vi "CLC_L2_8x8_InPhaseCal_L1_2x2.vi"() -> ()   [LabVIEW 2023, in "Clover_Cell.lvlib"]
uses:
  lib/CTL/AiP_index.ctl
  Clover_Cell.lvlib
  lib/Anritsu Signal Analyzer Series/Anritsu Signal Analyzer Series.lvlib
panel:
  out "output cluster 2":T1
  out "maxPower":dbl
  out "B_Ch_Index":i32[](array[numeric])
  out "A_Ch_Index":i32[](array[numeric])
  out "A-Phase":i32[](array[numeric])
  out "B-Phase":i32[](array[numeric])
  out "Duration(sec)":dbl
  out "Start":u32
  in  "AiP_Change":T2=1 items=["AiP_1"=1, "AiP_2"=2, "AiP_3"=3, "AiP_4"=4, "AiP_5"=5, "AiP_6"=6, "AiP_7"=7, "AiP_8"=8, "AiP_9"=9, "AiP_10"=10, "AiP_11"=11, "AiP_12"=12, "AiP_13"=13, "AiP_14"=14, "AiP_15"=15, "AiP_16"=16]
  in  "AiP_Base":T2=7 items=["AiP_1"=1, "AiP_2"=2, "AiP_3"=3, "AiP_4"=4, "AiP_5"=5, "AiP_6"=6, "AiP_7"=7, "AiP_8"=8, "AiP_9"=9, "AiP_10"=10, "AiP_11"=11, "AiP_12"=12, "AiP_13"=13, "AiP_14"=14, "AiP_15"=15, "AiP_16"=16]
  in  "WaitingTime":u32=500
  in  "Polarity":u16(ring) items=["H", "V"]
  in  "AvgTimes":i32=5
  in  "TRXmode":u16(ring)=1 items=["Rx"=2, "Tx"=1]
  in  "FileName_Note":string
  out "AiP_Base_Ch":i32
  out "AiP_Change_OFFSetPhase":i32
  out "AiP_Change_Ch":i32
  out "max index\n(OFFSet Step)":i32
  out "trmode":u16
  in  "VISA resource name":refnum<visa-resource-name>="TCPIP0::192.168.100.230::inst0::INSTR"
  out "FileNAME_Dual":string
  out "OK?":bool
  out "output cluster":T3={"address"="192.168.100.111", "remote port or service name"=5025, "timeout ms (60000)"=10000}
  out "SA1":dbl[](graph)
  out "error out":errorcluster
  # "CLC_Gen3_L2_8x8_InPhase_Calibration_by_L1_2x2"
  # "Setting"
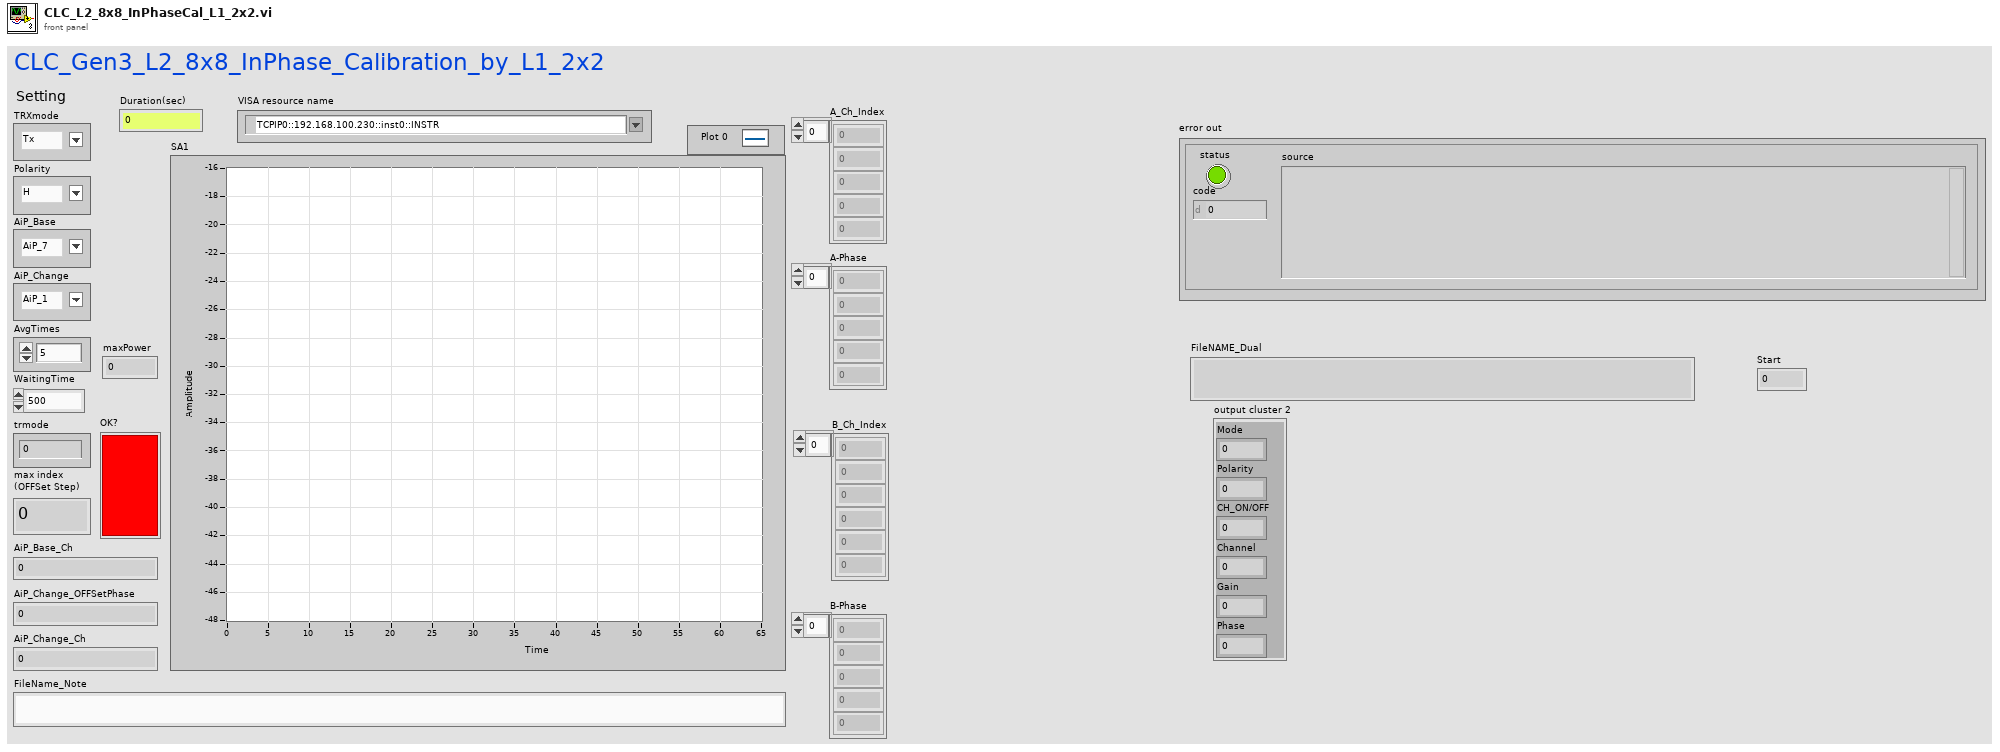
[diagram p1: front panel]
types:
  T1 = cluster{"Mode":u16, "Polarity":u16, "CH_ON/OFF":u16, "Channel":i32, "Gain":i32, "Phase":i32}
  T2 = typedef "AiP_index.ctl" = u16
  T3 = cluster{"address":string, "remote port or service name":u16, "timeout ms (60000)":i32}
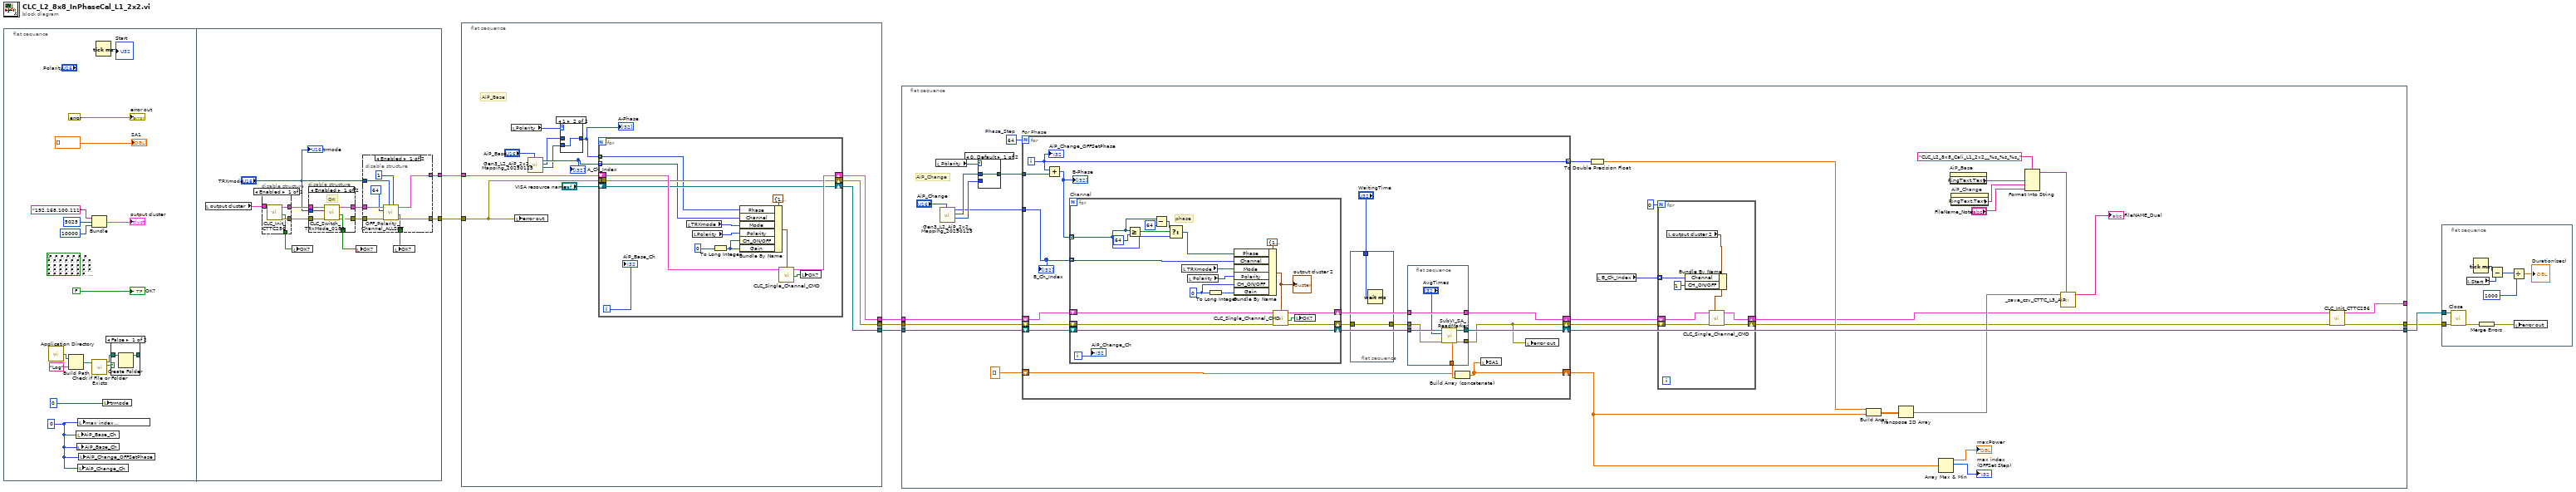
[diagram p0: block diagram]
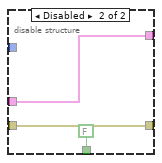
[diagram p5: hidden frame]
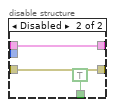
[diagram p6: hidden frame]
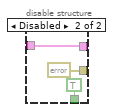
[diagram p7: hidden frame]
diagram:
  n1 = flat-sequence {
    tunnel: [w26] -> w1
    tunnel: [w31] -> w2
    frame #0 {
      w9 = 0 ("max index\n(OFFSet Step)")
      (unwired) bool[][] [[FALSE, FALSE, FALSE, FALSE, FALSE, FALSE, FALSE, FALSE], [FALSE, FALSE, FALSE, FALSE, FALSE, FALSE, FALSE, FALSE], [FALSE, FALSE, FALSE, FALSE, FALSE, FALSE, FALSE, FALSE], [FALSE, FALSE, FALSE, FALSE, FALSE, FALSE, FALSE, FALSE], [FALSE, FALSE, FALSE, FALSE, FALSE, FALSE, FALSE, FALSE], [FALSE, FALSE, FALSE, FALSE, FALSE, FALSE, FALSE, FALSE], [FALSE, FALSE, FALSE, FALSE, FALSE, FALSE, FALSE, FALSE], [FALSE, FALSE, FALSE, FALSE, FALSE, FALSE, FALSE, FALSE]] ("Operating \nChannel(s)")
      n2 = call <vilib>:"Application Directory.vi"() -> ("Application Directory"=w14:path)
      n3 = Build Path(base path=w14, name or relative path="Log") -> (appended path=w11:path)
      n4 = local write "AiP_Base_Ch"(w9) -> ()
      n5 = local write "AiP_Base_Ch"(w9) -> ()
      n6 = local write "AiP_Change_Ch"(w9) -> ()
      n7 = local write "max index\n(OFFSet Step)"(w9) -> ()
      n8 = local write "AiP_Change_OFFSetPhase"(w9) -> ()
      n9 = Bundle("address"="192.168.100.111", "remote port or service name"=u16 5025, "timeout ms (60000)"=10000) -> (→"output cluster":T3)  [unwired: 1 in]
      n10 = call <vilib>:"Check if File or Folder Exists.vi"("path"=w11) -> ("file or folder exists?"=w13:bool, "dup path"=w12:path)  [unwired: 8 in, 1 out]
      n11 = Tick Count (ms)() -> (millisecond timer value=→"Start":u32)
      n12 = local write "trmode"(u16 0 ("trmode")) -> ()
      n13 = case shown="False" w13 {
        tunnel: w12 -> [w24 w25]
        tunnel: [w23 w25] -> _
        frame False {
          n14 = Create Folder(path (use dialog)=w24) -> (created path=w23:path)  [unwired: 2 in, 2 out]
        }
        frame True {
        }
      }
      "error out" <- errorcluster {"status"=FALSE, "code"=0, "source"=""} ("error out")
      "OK?" <- FALSE ("OK?")
      "SA1" <- dbl[] []
    }
    frame #1 {
      n15 = local read "output cluster"() -> (w36:T3)
      n16 = disable-structure shown="Enabled" {
        disable-tunnel: w36 -> [w60 w63]
        disable-tunnel: [w59 w63] -> w35
        disable-tunnel: [w58 errorcluster {"status"=FALSE, "code"=0, "source"=""} ("error in (no error)")] -> w33
        disable-tunnel: [w57 TRUE ("OK?")] -> w28
        frame Enabled {
          n17 = call "CLC_Init_CTTC256.vi"("TCPIPin"=w60) -> ("error out"=w58:errorcluster, "Status"=w57:bool, "TCPIPin 2"=w59:T3)  [unwired: 8 in]
        }
        frame Disabled {
        }
      }
      n18 = local write "OK?"(w28) -> ()
      n19 = disable-structure shown="Enabled" {
        disable-tunnel: w35 -> [w53 w55]
        disable-tunnel: [w52 TRUE ("OK?")] -> w34
        disable-tunnel: w33 -> [w51 w54]
        disable-tunnel: [w50 w54] -> w32
        disable-tunnel: [w49 w55] -> w30
        disable-tunnel: "TRXmode" -> [w48 _]
        frame Enabled {
          # "OK"
          n20 = call "CLC_Switch_TRxMode_0188.vi"("error in (no error)"=w51, "Text Ring"=w48, "TCPIPin"=w53) -> ("error out"=w50:errorcluster, "OK?"=w52:bool, "TCPIPin 2"=w49:T3)  [unwired: 6 in]
        }
        frame Disabled {
        }
      }
      n21 = local write "OK?"(w34) -> ()
      n22 = disable-structure shown="Enabled" {
        disable-tunnel: w32 -> [w44 w46]
        disable-tunnel: [w43 w46] -> w31
        disable-tunnel: w30 -> [w42 w45]
        disable-tunnel: [w41 FALSE ("OK?")] -> w29
        disable-tunnel: "TRXmode" -> [w39 _]
        disable-tunnel: [w37 w45] -> w26
        frame Enabled {
          n23 = call "OFF_Polarity_Channel_ALLSET.vi"("CH_ON:0/OFF:1"=u16 1, "Mode"=w39, "error in"=w44, "Channel"=64, "TCPIPin"=w42) -> ("error out"=w43:errorcluster, "OK?"=w41:bool, "TCPIPout"=w37:T3)  [unwired: 4 in]
        }
        frame Disabled {
        }
      }
      n24 = local write "OK?"(w29) -> ()
      "trmode" <- "TRXmode"
    }
  }
  n25 = flat-sequence {
    tunnel: [w75] -> w7
    tunnel: [w74] -> w6
    tunnel: [w73] -> w5
    tunnel: w2 -> [w72]
    tunnel: w1 -> [w70]
    frame #0 {
      # "AiP_Base"
      n26 = local read "Polarity"() -> (w69:u16)
      n27 = local write "error out"(w72) -> ()
      n28 = call "Gen3_L2_AiP_2x2_Mapping_20250125.vi"("AiP"="AiP_Base") -> ("Pol_V"=w66:i32[], "Pol_H"=w67:i32[], "Ch_Index"=w68:i32[])  [unwired: 8 in]
      "A_Ch_Index" <- w68
      n29 = case shown="1" w69 {
        tunnel: w67 -> [w76 _]
        tunnel: [w76 w77] -> w64
        tunnel: w66 -> [_ w77]
        frame 0, Default {
        }
        frame 1 {
        }
      }
      "A-Phase" <- w64
      n30 = for {
        shift-right: [w88] -> w73
        shift-left: w70 -> [w87]
        tunnel: w72 -> [w82]
        shift-right: [w82] -> w74
        shift-left: _ -> [_]
        shift-right: [w81] -> w75
        shift-left: "VISA resource name" -> [w81]
        tunnel: w68 -> [w80] mode=indexing
        tunnel: w64 -> [w79] mode=indexing
        i -> [w78]
        n31 = local read "TRXmode"() -> (w85:u16)
        n32 = local read "Polarity"() -> (w84:u16)
        n33 = To Long Integer(number=u16 0 ("CH_ON/OFF")) -> (32bit integer=w83:i32)
        n34 = Bundle By Name(cluster=T1 {"Mode"=1, "Polarity"=1, "CH_ON/OFF"=1, "Channel"=0, "Gain"=0, "Phase"=0} ("Channel params"), "Phase"=w79, "Channel"=w80, "Mode"=w85, "Polarity"=w84, "CH_ON/OFF"=w83, "Gain"=w83) -> (w91:T1)
        n35 = call "CLC_Single_Channel_CMD.vi"("Channel params"=w91, "TCPIPin"=w87) -> ("OK?"=w90:bool, "TCPIPout"=w88:T3)  [unwired: 7 in, 1 out]
        n36 = local write "OK?"(w90) -> ()
        "AiP_Base_Ch" <- w78
      }
    }
  }
  n37 = flat-sequence {
    tunnel: w7 -> [w124]
    tunnel: w6 -> [w123]
    tunnel: w5 -> [w122]
    tunnel: [w120] -> w4
    tunnel: [w107] -> w3
    tunnel: [w108] -> _
    frame #0 {
      w119 = 64  # Phase_Step
      # "AiP_Change"
      n38 = local read "Polarity"() -> (w117:u16)
      n39 = call "Gen3_L2_AiP_2x2_Mapping_20250125.vi"("AiP"="AiP_Change") -> ("Pol_V"=w115:i32[], "Pol_H"=w116:i32[], "Ch_Index"=w114:i32[])  [unwired: 8 in]
      n40 = case shown="0, Default" w117 {
        tunnel: w116 -> [w133 _]
        tunnel: [w133 w134] -> w113
        tunnel: w115 -> [_ w134]
        frame 0, Default {
        }
        frame 1 {
        }
      }
      n41 = for "For Phase" {
        N: w119 -> [_]
        shift-right: [w146] -> w96
        shift-left: w122 -> [w148]
        shift-right: [w145] -> w97
        shift-left: w123 -> [w149]
        shift-right: [w152] -> w120
        shift-left: w124 -> [w143]
        shift-right: [w147] -> w112
        shift-left: dbl[] [] -> [w150]
        tunnel: w114 -> [w141]
        tunnel: w113 -> [w140]
        tunnel: [w138] -> w110 mode=indexing
        i -> [w138]
        n42 = Add(x=w138, y=w140) -> (x+y=w139:i32[])
        "B-Phase" <- w139
        n43 = for "Channel" {
          shift-right: [w164] -> w137
          shift-left: w149 -> [w169]
          shift-right: [w165] -> w144
          shift-left: w148 -> [w168]
          shift-right: [w163] -> w142
          shift-left: w143 -> [w163]
          tunnel: w141 -> [w162] mode=indexing
          tunnel: w139 -> [w157] mode=indexing
          i -> [w155]
          w173 = u16 0 ("CH_ON/OFF")
          # "phase"
          n44 = Greater Or Equal?(x=w157, y=64) -> (x >= y?=w160:bool)
          n45 = Subtract(x=w157, y=64) -> (x-y=w161:i32)
          n46 = Select(t=w161, s=w160, f=w157) -> (s? t:f=w156:i32)
          n47 = local read "TRXmode"() -> (w171:u16)
          n48 = local read "Polarity"() -> (w172:u16)
          n49 = To Long Integer(number=w173) -> (32bit integer=w174:i32)
          n50 = Bundle By Name(cluster=T1 {"Mode"=1, "Polarity"=1, "CH_ON/OFF"=1, "Channel"=0, "Gain"=0, "Phase"=0} ("Channel params"), "Phase"=w156, "Channel"=w162, "Mode"=w171, "Polarity"=w172, "CH_ON/OFF"=w173, "Gain"=w174) -> (w166:T1)
          "output cluster 2" <- w166
          n51 = call "CLC_Single_Channel_CMD.vi"("Channel params"=w166, "error in"=w169, "TCPIPin"=w168) -> ("error out"=w164:errorcluster, "OK?"=w167:bool, "TCPIPout"=w165:T3)  [unwired: 6 in]
          n52 = local write "OK?"(w167) -> ()
          "AiP_Change_Ch" <- w155
        }
        n53 = flat-sequence {
          tunnel: w137 -> [w154]
          tunnel: [w154] -> w136
          tunnel: "WaitingTime" -> [w153]
          frame #0 {
            n54 = Wait (ms)(milliseconds to wait=w153) -> ()  [unwired: 1 out]
          }
        }
        n55 = flat-sequence {
          tunnel: [w181] -> w152
          tunnel: [w180] -> w151
          tunnel: [w179] -> w145
          tunnel: w142 -> [w178]
          tunnel: w136 -> [w177]
          tunnel: [w176] -> w146
          tunnel: w144 -> [w176]
          frame #0 {
            n56 = call "SubVI_SA_ReadMarker.vi"("error in (no error)"=w177, "AvgTimes"="AvgTimes", "VISA resource name"=w178) -> ("error out"=w179:errorcluster, "VISA resource name out"=w181:refnum<visa-resource-name>, "Marker Power"=w180:dbl)  [unwired: 5 in, 1 out]
          }
        }
        n57 = Build Array (concatenate)(w150, w151) -> (w147:dbl[])
        n58 = local write "SA1"(w147) -> ()
        n59 = local write "error out"(w145) -> ()
        "AiP_Change_OFFSetPhase" <- w138
        "B_Ch_Index" <- w141
      }
      n60 = To Double Precision Float(number=w110) -> (double precision float=w109:dbl[])
      n61 = local read "B_Ch_Index"() -> (w92:i32[])
      n62 = for {
        N: 0 -> [_]
        shift-right: [w129] -> w95
        shift-left: w96 -> [w130]
        shift-right: [w131] -> w94
        shift-left: w97 -> [w132]
        tunnel: w92 -> [w126] mode=indexing
        n63 = local read "output cluster 2"() -> (w127:T1)
        n64 = Bundle By Name(cluster=w127, "Channel"=w126, "CH_ON/OFF"=u16 1) -> (w128:T1)
        n65 = call "CLC_Single_Channel_CMD.vi"("Channel params"=w128, "error in"=w132, "TCPIPin"=w130) -> ("error out"=w131:errorcluster, "TCPIPout"=w129:T3)  [unwired: 6 in, 1 out]
      }
      n66 = Build Array(w109, w112) -> (w121:dbl[][])
      n67 = Transpose 2D Array(2D array=w121) -> (transposed array=w98:dbl[][])
      n68 = Array Max & Min(array=w112) -> (max value=→"maxPower":dbl, max index (indices)=→"max index\n(OFFSet Step)":i32)  [unwired: 2 out]
      n69 = property on="AiP_Base" class="Ring (strict)"() -> ("RingText.Text"=w102:string)  [unwired: 2 in, 2 out]
      n70 = property on="AiP_Change" class="Ring (strict)"() -> ("RingText.Text"=w103:string)  [unwired: 2 in, 2 out]
      n71 = Format Into String(format string="CLC_L2_8x8_Cali_L1_2x2__%s_%s_%s_", w102, w103, "FileName_Note") -> (resulting string=w101:string)  [unwired: 2 in, 1 out]
      n72 = call "_save_csv_CTTC_L3_AiP.vi"("delimiter (\\t)"=w101, "Data"=w98) -> ("FileName"=→"FileNAME_Dual":string)  [unwired: 9 in]
      n73 = call "CLC_Init_CTTC256.vi"("error in (no error)"=w94, "TCPIPin"=w95) -> ("error out"=w107:errorcluster, "TCPIPin 2"=w108:T3)  [unwired: 7 in, 1 out]
    }
  }
  n74 = flat-sequence {
    tunnel: w4 -> [w189]
    tunnel: w3 -> [w188]
    frame #0 {
      n75 = call "Close.vi"("error in (no error)"=w188, "VISA resource name"=w189) -> ("error out"=w190:errorcluster)  [unwired: 9 in]
      n76 = local read "Start"() -> (w185:u32)
      n77 = Tick Count (ms)() -> (millisecond timer value=w186:u32)
      n78 = Merge Errors(w190) -> (w187:errorcluster)
      n79 = Subtract(x=w186, y=w185) -> (x-y=w184:u32)
      n80 = Divide(x=w184, y=u32 1000) -> (x/y=→"Duration(sec)":dbl)
      n81 = local write "error out"(w187) -> ()
    }
  }
